vi "Main.vi"() -> ()   [LabVIEW 2017]
doc: "The myRIO Project template acquires acceleration data from the onboard accelerometer and displays the changes of acceleration values in a waveform chart."
uses:
  <vilib>/myRIO/Instrument Drivers/Onboard IO/AI/typedefs/AI Reference.ctl
  <vilib>/myRIO/Common/Instrument Driver Framework/Utilities/typedefs/myRIO Generic Hardware Reference.ctl
  <vilib>/myRIO/Common/Instrument Driver Framework/Utilities/typedefs/Hardware Version Enum.ctl
  <vilib>/myRIO/Common/Instrument Driver Framework/Utilities/typedefs/myRIO v1.0 Reference.ctl
  <vilib>/myRIO/Common/Instrument Driver Framework/Utilities/typedefs/Generic FPGA Reference.ctl
  <vilib>/myRIO/Common/Instrument Driver Framework/myRIO v1.0/AI/typedefs/AI Channels List.ctl
  <vilib>/myRIO/Common/Instrument Driver Framework/myRIO v1.0/AI/typedefs/AI Channels Enum.ctl
  <vilib>/myRIO/Common/Instrument Driver Framework/Utilities/typedefs/Analog Scaling Constants List.ctl
  <vilib>/myRIO/Common/Instrument Driver Framework/Utilities/typedefs/Analog Scaling Constants.ctl
  <vilib>/userdefined/High Color/nirio_resource_hc.ctl
  <vilib>/myRIO/Instrument Drivers/Onboard IO/DIO/typedefs/DIO Reference.ctl
  <vilib>/myRIO/Common/Instrument Driver Framework/myRIO v1.0/DIO/typedefs/DIO Channels List.ctl
  <vilib>/myRIO/Common/Instrument Driver Framework/myRIO v1.0/DIO/typedefs/DIO Channels Enum.ctl
  <vilib>/myRIO/Common/Instrument Driver Framework/Utilities/vis/Is FPGA Ref Available.vi
  <vilib>/myRIO/Common/Instrument Driver Framework/myRIO v1.0/DIO/vis/myRIO v1.1 Open DIO.vi
  <vilib>/myRIO/Instrument Drivers/Onboard IO/DIO/vis/Write.vi
  <vilib>/myRIO/Common/Instrument Driver Framework/myRIO v1.0/AI/vis/myRIO v1.1 Open AI.vi
  <vilib>/myRIO/Instrument Drivers/Onboard IO/AI/vis/Read.vi
  <vilib>/myRIO/Common/Instrument Driver Framework/Utilities/vis/Validate Channels.vi
  <vilib>/myRIO/Common/Instrument Driver Framework/myRIO v1.0/DIO/vis/myRIO v1.0 Reserve DIO.vi
  <vilib>/myRIO/Common/Instrument Driver Framework/myRIO v1.0/AI/vis/myRIO v1.0 Reserve AI.vi
  <vilib>/myRIO/Common/Instrument Driver Framework/myRIO v1.0/Resource Manager/vis/myRIO v1.0 Reserve Channel List.vi
  <vilib>/myRIO/Common/Instrument Driver Framework/myRIO v1.0/DIO/vis/myRIO v1.0 Build MUX Configuration DIO.vi
  <vilib>/myRIO/Common/Instrument Driver Framework/myRIO v1.0/AI/vis/myRIO v1.0 Build MUX Configuration AI.vi
  <vilib>/myRIO/Common/Instrument Driver Framework/myRIO v1.0/Resource Manager/vis/myRIO v1.0 Reserve Channel.vi
  <vilib>/myRIO/Common/Instrument Driver Framework/myRIO v1.0/Resource Manager/vis/myRIO v1.0 Unreserve Channel.vi
  <vilib>/myRIO/Common/Instrument Driver Framework/myRIO v1.0/Resource Manager/vis/myRIO v1.0 Create Configuration List.vi
  <vilib>/myRIO/Common/Instrument Driver Framework/myRIO v1.0/Resource Manager/vis/myRIO v1.0 Build Mutex Name.vi
  GlobalVar.vi
  <vilib>/Utility/VariantDataType/GetNumericInfo.vi
  <vilib>/Utility/error.llb/Error Cluster From Error Code.vi
  <vilib>/myRIO/Common/Instrument Driver Framework/myRIO v1.0/myRIO v1.1 Open.vi
  <vilib>/myRIO/Common/Instrument Driver Framework/myRIO v1.0/AI/vis/myRIO v1.0 Get Scaling Constants AI.vi
  <vilib>/myRIO/Common/Instrument Driver Framework/Utilities/vis/IO Manager.vi
  <vilib>/myRIO/Common/Instrument Driver Framework/Utilities/vis/Configuration Manager.vi
  <vilib>/myRIO/Common/Instrument Driver Framework/myRIO v1.0/myRIO v1.0 Close.vi
  <vilib>/myRIO/Common/Instrument Driver Framework/myRIO v1.0/AI/vis/myRIO v1.0 Read AI.vi
  <vilib>/myRIO/Common/Instrument Driver Framework/myRIO v1.0/Resource Manager/vis/myRIO v1.0 Configure IO.vi
  <vilib>/myRIO/Common/Instrument Driver Framework/myRIO v1.0/DIO/vis/myRIO v1.0 Write DIO.vi
  <vilib>/myRIO/Express VI/Onboard IO/AI/AI Express VI.xnode
  <vilib>/myRIO/Instrument Drivers/Onboard IO/AI/vis/myRIO AI Open.xnode
  <vilib>/myRIO/Express VI/Onboard Devices/LED/LED Express VI.xnode
  <vilib>/myRIO/Instrument Drivers/Onboard IO/DIO/vis/myRIO DIO Open.xnode
  <vilib>/myRIO/Instrument Drivers/Onboard IO/AI/AI.lvlib
  <vilib>/myRIO/Instrument Drivers/Onboard IO/DIO/DIO.lvlib
  <vilib>/myRIO/Express VI/Onboard Devices/Button/Button Express VI.xnode
  <vilib>/myRIO/Instrument Drivers/Onboard IO/DIO/vis/Read.vi
panel:
  in  "x":dbl
  in  "Stop Button 2":bool
  in  "Stop (F)":bool
  out "Image Out":T1(plugin-control)
  in  "Carzeta":dbl
  in  "Stop Button":bool
  out "lb (B/AI3 (Pin 9))":dbl
  out "lf (B/AI2 (Pin 7))":dbl
  out "r (B/AI1 (Pin 5))":dbl
  out "l (B/AI0 (Pin 3))":dbl
  out "L_MOTOR_POS":i32
  out "R_MOTOR_POS":i32
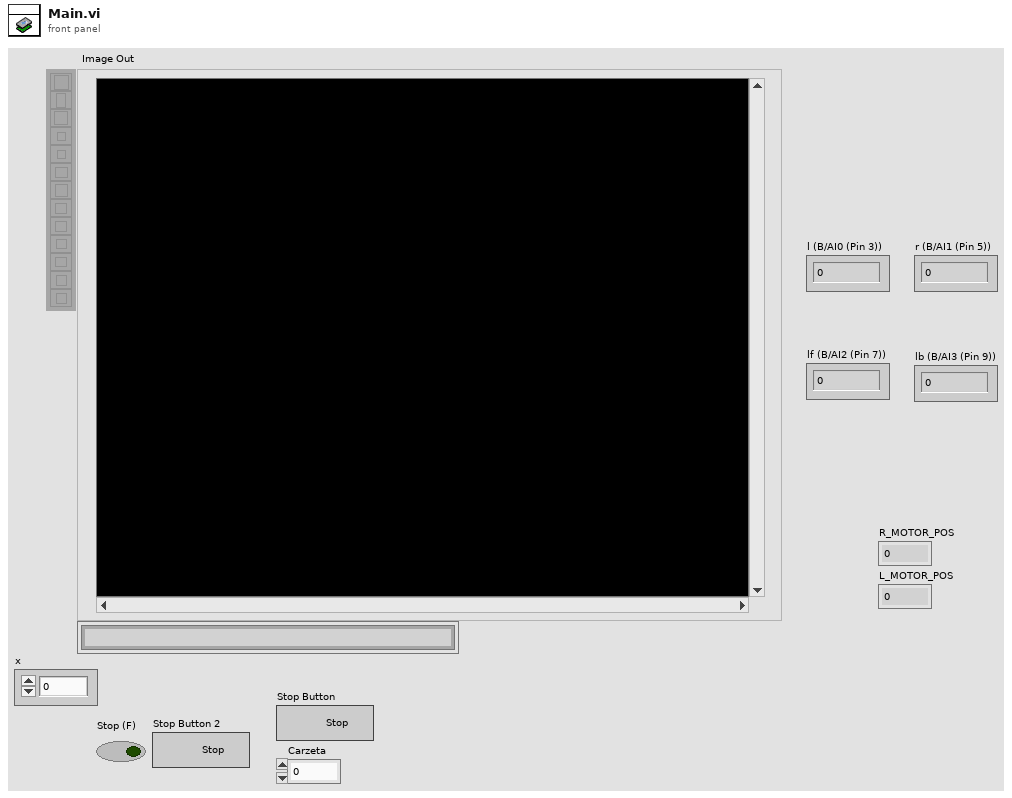
[diagram p1: front panel]
types:
  T1 = typedef "IMAQ Image.ctl" = refnum<image>
  T2 = typedef "AI.lvlib/AI Reference.ctl" = cluster{"myRIO Reference":T3, "AI Channels List":T7, "AI Scaling Constants List":T9}
  T3 = typedef "myRIO Generic Hardware Reference.ctl" = cluster{"myRIO Model":T4, "myRIO Hardware Reference":T5}
  T4 = typedef "Hardware Version Enum.ctl" = enum16{"Unknown", "myRIO-1900", "myRIO-1950", "roboRIO", "NI ELVIS RIO CM"}
  T5 = typedef "myRIO v1.0 Reference.ctl" = cluster{"Generic FPGA Reference":T6, "Allow multiple opens":bool}
  T6 = typedef "Generic FPGA Reference.ctl" = refnum<k20>
  T7 = typedef "AI Channels List.ctl" = T8[]
  T8 = typedef "AI Channels Enum.ctl" = enum16{"Not Connected", "AudioIn/Left", "AudioIn/Right", "C/AI0", "C/AI1", "A/AI0", "A/AI1", "A/AI2", "A/AI3", "B/AI0", "B/AI1", "B/AI2", "B/AI3", "AI/AI0", "AI/AI1", "AI/AI2", "AI/AI3"}
  T9 = typedef "Analog Scaling Constants List.ctl" = T10[]
  T10 = typedef "Analog Scaling Constants.ctl" = cluster{"LSB Weight (Volts)":dbl, "Offset (Volts)":dbl, "Signed?":bool}
  T11 = typedef "nirio_resource_hc.ctl" = tag
  T12 = typedef "DIO.lvlib/DIO Reference.ctl" = cluster{"myRIO Reference":T3, "DIO Channels List":T13}
  T13 = typedef "DIO Channels List.ctl" = T14[]
  T14 = typedef "DIO Channels Enum.ctl" = enum16{"Not Connected", "C/DIO0", "C/DIO1", "C/DIO2", "C/DIO3", "C/DIO4", "C/DIO5", "C/DIO6", "C/DIO7", "A/DIO0", "A/DIO1", "A/DIO2", "A/DIO3", "A/DIO4", "A/DIO5", "A/DIO6", "A/DIO7", "A/DIO8", "A/DIO9", "A/DIO10", "A/DIO11", "A/DIO12", "A/DIO13", "A/DIO14", "A/DIO15", "B/DIO0", "B/DIO1", "B/DIO2", "B/DIO3", "B/DIO4", "B/DIO5", "B/DIO6", "B/DIO7", "B/DIO8", "B/DIO9", "B/DIO10", "B/DIO11", "B/DIO12", "B/DIO13", "B/DIO14", "B/DIO15", "LED0", "LED1", "LED2", "LED3", "Button0", "DIO/DIO0", "DIO/DIO1", "DIO/DIO2", "DIO/DIO3", "DIO/DIO4", "DIO/DIO5", "DIO/DIO6", "DIO/DIO7", "DIO/DIO8", "DIO/DIO9", "SPI/CS0", "SPI/CS1", "SPI/CS2", "SPI/CS3", "LED RADIO (Green)", "LED RADIO (Red)", "LED COMM (Green)", "LED COMM (Red)", "LED MODE (Green)", "LED MODE (Red)"}
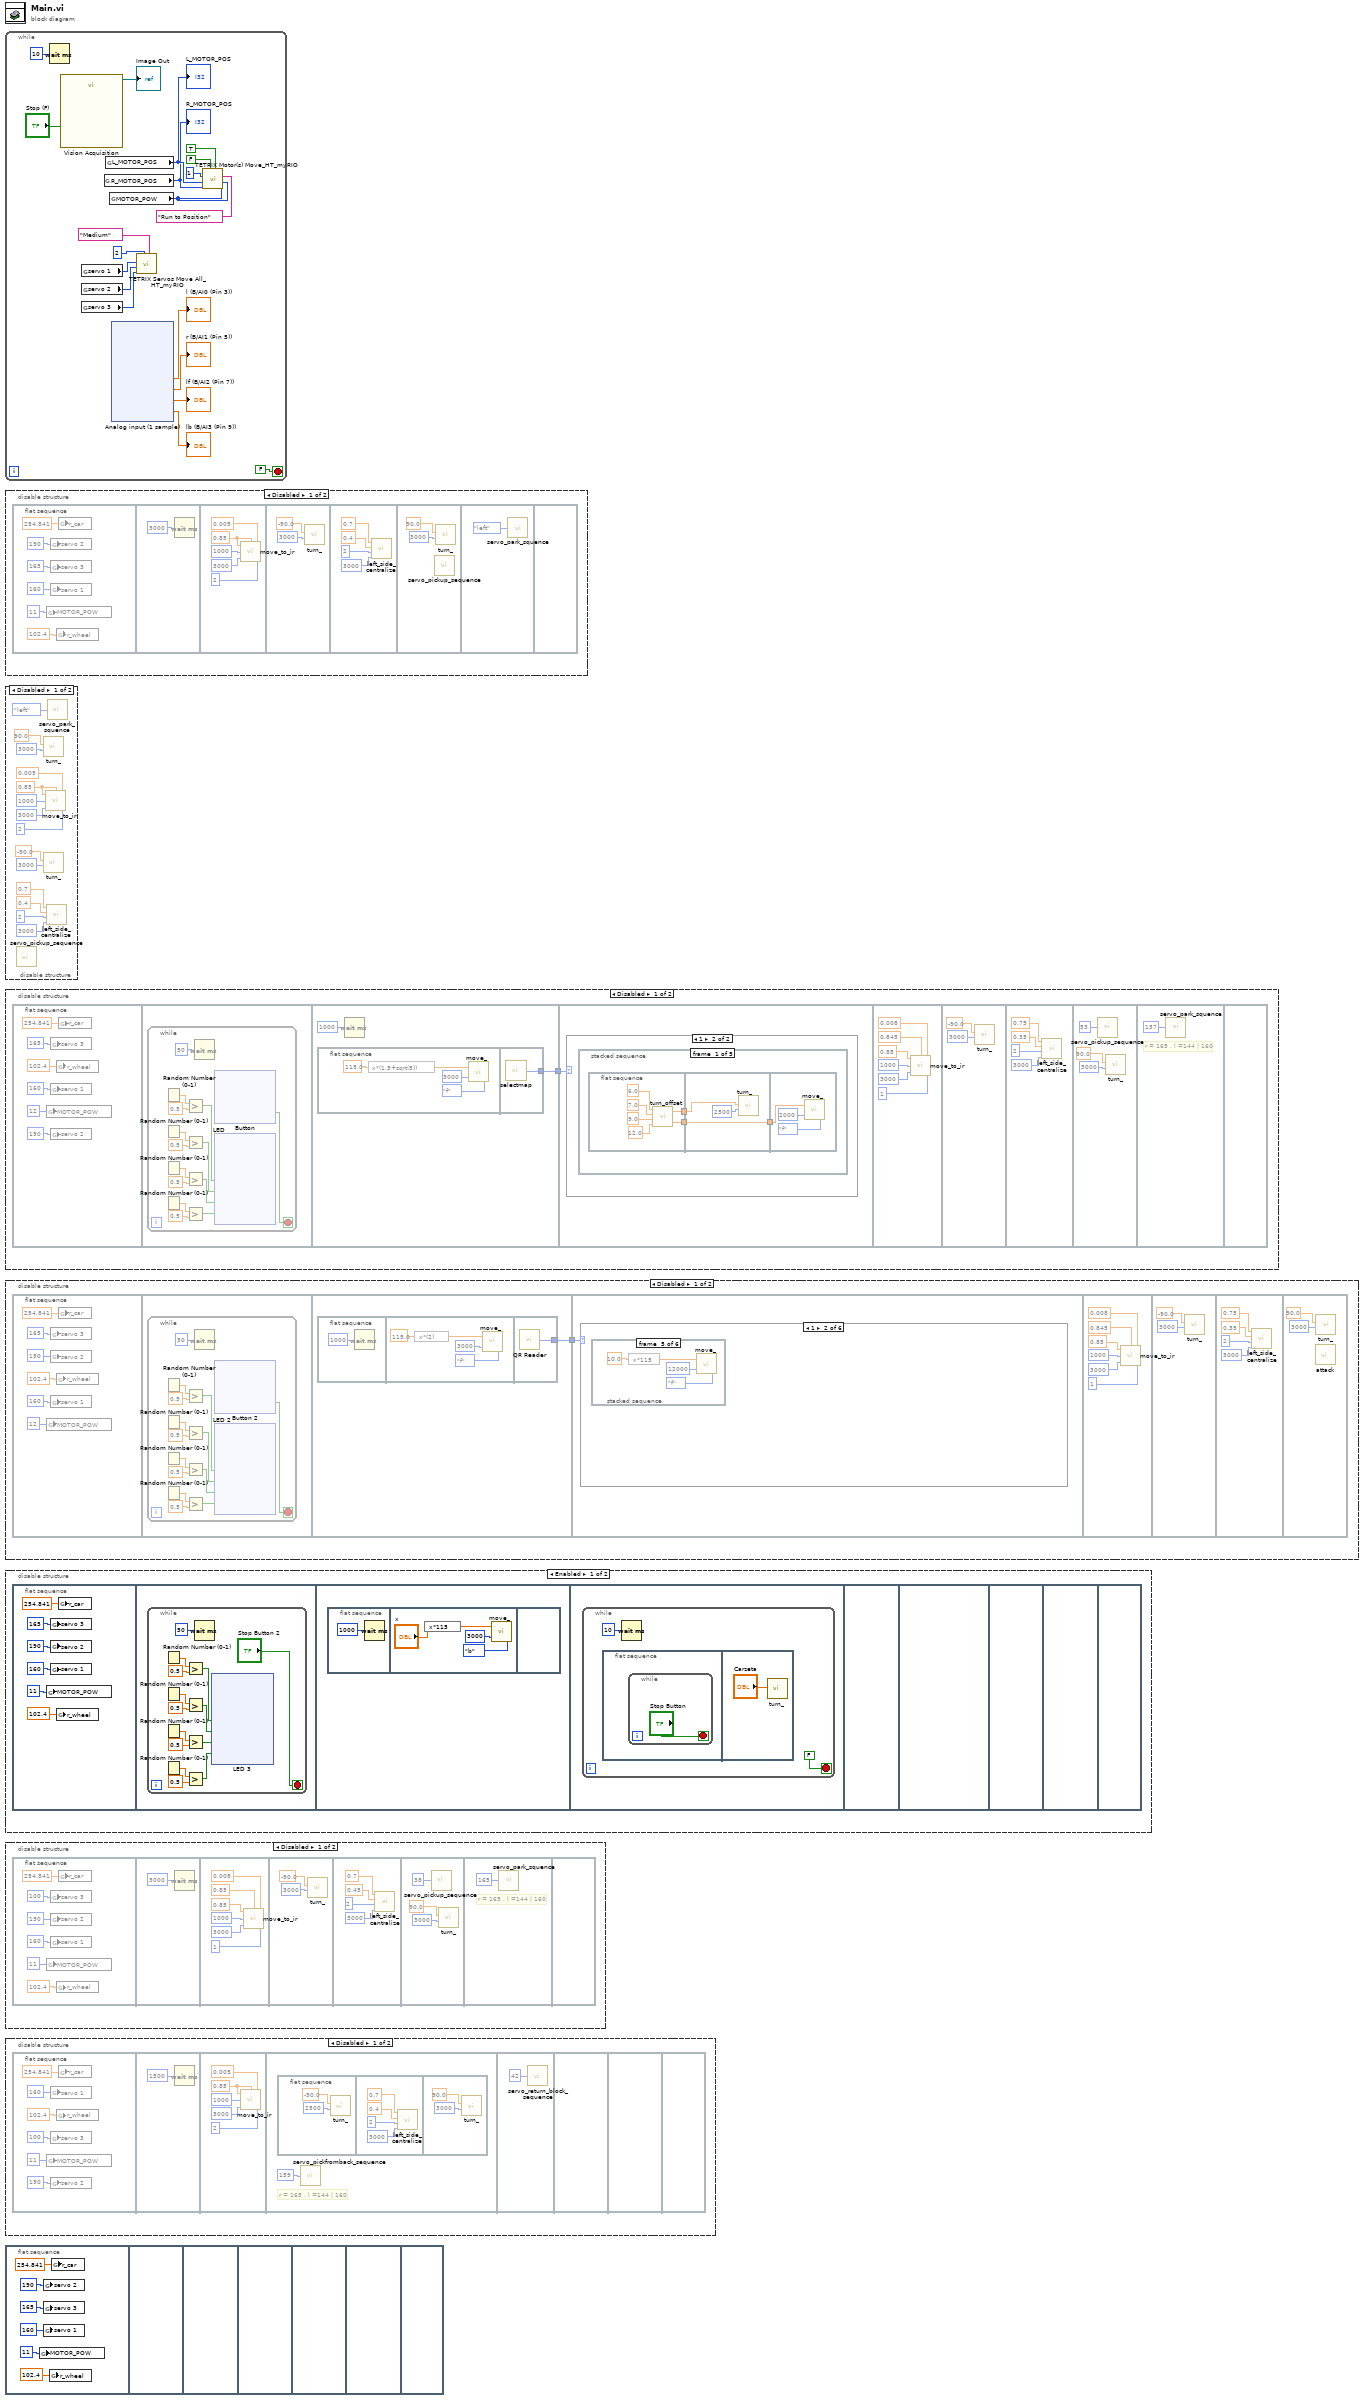
[diagram p0: block diagram]
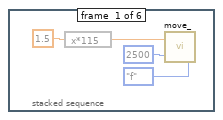
[diagram p3: hidden frame]
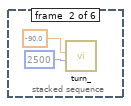
[diagram p4: hidden frame]
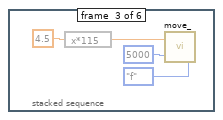
[diagram p5: hidden frame]
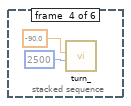
[diagram p6: hidden frame]
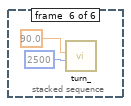
[diagram p7: hidden frame]
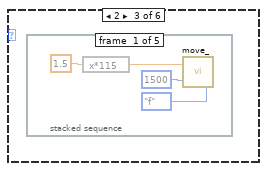
[diagram p8: hidden frame]
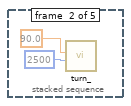
[diagram p9: hidden frame]
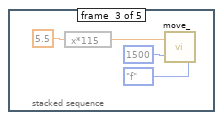
[diagram p10: hidden frame]
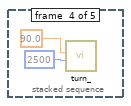
[diagram p11: hidden frame]
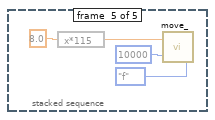
[diagram p12: hidden frame]
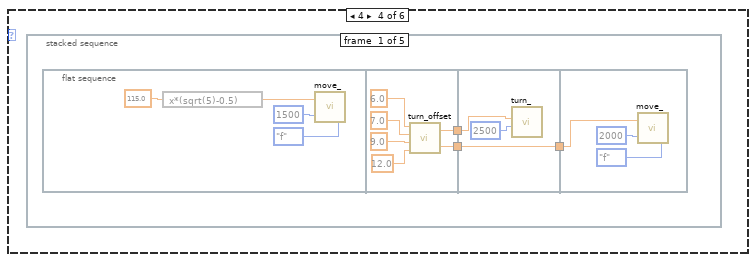
[diagram p13: hidden frame]
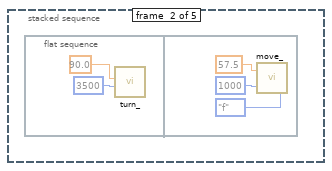
[diagram p14: hidden frame]
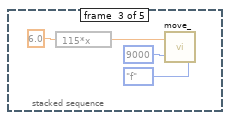
[diagram p15: hidden frame]
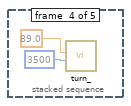
[diagram p16: hidden frame]
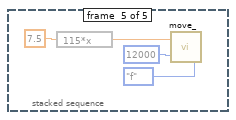
[diagram p17: hidden frame]
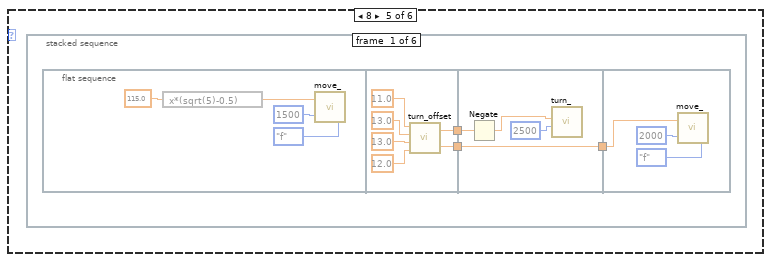
[diagram p18: hidden frame]
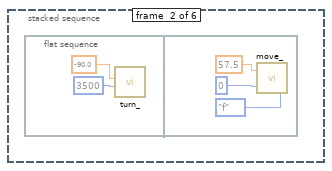
[diagram p19: hidden frame]
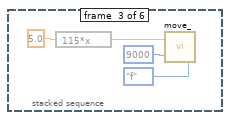
[diagram p20: hidden frame]
diagram:
  n1 = while {
    stop <- FALSE stop-if-true
    n2 = Wait (ms)(milliseconds to wait=u32 10) -> ()  [unwired: 1 out]
    n3 = call "Vision Acquisition"("Stop (F)"="Stop (F)") -> ("Image Out"=→"Image Out":T1)  [unwired: 24 in, 2 out]
    n4 = global read "GlobalVar.vi" "servo 1"() -> (w5:u8)
    n5 = global read "GlobalVar.vi" "servo 2"() -> (w4:u8)
    n6 = global read "GlobalVar.vi" "servo 3"() -> (w3:u8)
    n7 = global read "GlobalVar.vi" "R_MOTOR_POS"() -> (w13:i32)
    "R_MOTOR_POS" <- w13
    n8 = global read "GlobalVar.vi" "L_MOTOR_POS"() -> (w14:i32)
    "L_MOTOR_POS" <- w14
    n9 = global read "GlobalVar.vi" "MOTOR_POW"() -> (w15:i8)
    n10 = xnode "Analog input (1 sample)"() -> ("l (B/AI0 (Pin 3))"=→"l (B/AI0 (Pin 3))":dbl, "r (B/AI1 (Pin 5))"=→"r (B/AI1 (Pin 5))":dbl, "lf (B/AI2 (Pin 7))"=→"lf (B/AI2 (Pin 7))":dbl, "lb (B/AI3 (Pin 9))"=→"lb (B/AI3 (Pin 9))":dbl)  [unwired: 1 in, 1 out]
    n11 = call <vilib>:"TETRIX Servos Move All_HT_myRIO.vi"("Enable Sync: Fast | Medium | Slow | None"="Medium", "Controller Daisy Chain Position (1 - 4)"=u8 2, "Servo 3 (0 - 255)"=w3, "Servo 2 (0 - 255)"=w4, "Servo 1 (0 - 255)"=w5) -> ()  [unwired: 4 in, 1 out]
    n12 = call <vilib>:"TETRIX Motor(s) Move_HT_myRIO.vi"("Motor 2 Power (-100 to 100)\n0 = Stop/Brake\n-128 = Stop/Coast"=w15, "Motor 1 Power (-100 to 100)\n0 = Stop/Brake\n-128 = Stop/Coast"=w15, "Control Mode"="Run to Position", "Motor 2 Reverse? : T or F"=TRUE, "Motor 1 Reverse? : T or F"=FALSE, "Encoder 2 Target: 360 = 1 motor shaft revolution"=w13, "Encoder 1 Target: 360 = 1 motor shaft revolution"=w14, "Controller Daisy Chain Position: 1 - 4"=u8 1) -> ()  [unwired: 1 in, 1 out]
  }
  n13 = disable-structure shown="Disabled" {
    frame Disabled {
      n14 = flat-sequence {
        frame #0 {
          n15 = global write "GlobalVar.vi" "MOTOR_POW"(i8 11 ("MOTOR_POW")) -> ()
          n16 = global write "GlobalVar.vi" "servo 2"(u8 190 ("servo 2")) -> ()
          n17 = global write "GlobalVar.vi" "servo 3"(u8 165 ("servo 3")) -> ()
          n18 = global write "GlobalVar.vi" "servo 1"(u8 160 ("servo 1")) -> ()
          n19 = global write "GlobalVar.vi" "r_wheel"(102.4 ("r_wheel")) -> ()
          n20 = global write "GlobalVar.vi" "r_car"(254.841 ("r_car")) -> ()
        }
        frame #1 {
          n21 = Wait (ms)(milliseconds to wait=u32 3000) -> ()  [unwired: 1 out]
        }
        frame #2 {
          w72 = 0.85 ("target_ir_r")
          n22 = call "move_to_ir.vi"("step"=2, "precision"=0.005, "target_ir_r"=w72, "samples"=3000, "delay_after"=u32 1000, "target_ir_l"=w72) -> ()
        }
        frame #3 {
          n23 = call "turn_.vi"("delay"=u32 3000, "Carzeta"=-90.0) -> ()  [unwired: 10 in]
        }
        frame #4 {
          n24 = call "left_side_centralize.vi"("samples"=3000, "step(mm)"=2, "inner_b_ir"=0.4, "inner_f_ir"=0.7) -> ()
        }
        frame #5 {
          n25 = call "servo_pickup_sequence.vi"() -> ()  [unwired: 12 in]
          n26 = call "turn_.vi"("delay"=u32 3000, "Carzeta"=90.0) -> ()  [unwired: 10 in]
        }
        frame #6 {
          n27 = call "servo_park_squence.vi"("servo 3"=enum16{"left", "right"}."left" ("pos")) -> ()
        }
        frame #7 {
        }
      }
    }
    frame Enabled {
    }
  }
  n28 = disable-structure shown="Disabled" {
    frame Disabled {
      w82 = 0.85 ("target_ir_r")
      n29 = call "servo_pickup_sequence.vi"() -> ()  [unwired: 1 in]
      n30 = call "turn_.vi"("delay"=u32 3000, "Carzeta"=90.0) -> ()  [unwired: 10 in]
      n31 = call "turn_.vi"("delay"=u32 3000, "Carzeta"=-90.0) -> ()  [unwired: 10 in]
      n32 = call "move_to_ir.vi"("step"=2, "precision"=0.005, "target_ir_r"=w82, "samples"=3000, "delay_after"=u32 1000, "target_ir_l"=w82) -> ()
      n33 = call "left_side_centralize.vi"("samples"=3000, "step(mm)"=2, "inner_b_ir"=0.4, "inner_f_ir"=0.7) -> ()
      n34 = call "servo_park_squence.vi"("servo 3"=enum16{"left", "right"}."left" ("pos")) -> ()
    }
    frame Enabled {
    }
  }
  n35 = disable-structure shown="Disabled" {
    frame Disabled {
      n36 = flat-sequence {
        tunnel: [w190] -> w96
        tunnel: w96 -> [w197]
        frame #0 {
          n37 = global write "GlobalVar.vi" "MOTOR_POW"(i8 12 ("MOTOR_POW")) -> ()
          n38 = global write "GlobalVar.vi" "servo 3"(u8 165 ("servo 3")) -> ()
          n39 = global write "GlobalVar.vi" "servo 1"(u8 160 ("servo 1")) -> ()
          n40 = global write "GlobalVar.vi" "servo 2"(u8 190 ("servo 2")) -> ()
          n41 = global write "GlobalVar.vi" "r_wheel"(102.4 ("r_wheel")) -> ()
          n42 = global write "GlobalVar.vi" "r_car"(254.841 ("r_car")) -> ()
        }
        frame #1 {
          n43 = while {
            stop <- w103 stop-if-true
            n44 = Random Number (0-1)() -> (number: 0 to 1=w108:dbl)
            n45 = Random Number (0-1)() -> (number: 0 to 1=w115:dbl)
            n46 = Random Number (0-1)() -> (number: 0 to 1=w112:dbl)
            n47 = Random Number (0-1)() -> (number: 0 to 1=w111:dbl)
            n48 = Greater?(x=w108, y=0.5) -> (0:w107:bool)
            n49 = Greater?(x=w115, y=0.5) -> (0:w106:bool)
            n50 = Greater?(x=w112, y=0.5) -> (0:w105:bool)
            n51 = Greater?(x=w111, y=0.5) -> (0:w104:bool)
            n52 = Wait (ms)(milliseconds to wait=u32 50) -> ()  [unwired: 1 out]
            n53 = xnode "Button"() -> ("Value"=w103:bool)  [unwired: 1 in, 1 out]
            n54 = xnode "LED"("LED0"=w107, "LED1"=w106, "LED2"=w105, "LED3"=w104) -> ()  [unwired: 1 in, 1 out]
          }
        }
        frame #2 {
          n55 = flat-sequence {
            tunnel: [w196] -> w190
            frame #0 {
              n56 = expression code="x*(1.5+sqrt(5))"(115.0 ("x")) -> (w195:dbl)
              n57 = call "move_.vi"("Enum"=enum16{"hold", "f", "b"}."f", "delay"=u32 3000, "D"=w195) -> ()  [unwired: 1 in]
            }
            frame #1 {
              n58 = call "selectmap.vi"() -> ("binary"=w196:u32)
            }
          }
          n59 = Wait (ms)(milliseconds to wait=u32 1000) -> ()  [unwired: 1 out]
        }
        frame #3 {
          n60 = case shown="1" w197 {
            frame 0, Default {
            }
            frame 1 {
              n61 = stacked-sequence {
                frame #0 {
                  n62 = flat-sequence {
                    tunnel: [w202] -> w200
                    tunnel: [w201] -> w198
                    tunnel: w200 -> [w208]
                    tunnel: [w207] -> w199
                    tunnel: w198 -> [w207]
                    tunnel: w199 -> [w210]
                    frame #0 {
                      n63 = call "turn_offset.vi"("x2"=12.0, "x1"=9.0, "y2"=7.0, "y1"=6.0) -> ("dis_"=w201:dbl, "zeta"=w202:dbl)
                    }
                    frame #1 {
                      n64 = call "turn_.vi"("delay"=u32 2500, "Carzeta"=w208) -> ()  [unwired: 10 in]
                    }
                    frame #2 {
                      n65 = call "move_.vi"("Enum"=enum16{"hold", "f", "b"}."f", "delay"=u32 2000, "D"=w210) -> ()  [unwired: 1 in]
                    }
                  }
                }
                frame #1 {
                  n66 = flat-sequence {
                    frame #0 {
                      n67 = call "turn_.vi"("delay"=u32 3500, "Carzeta"=90.0) -> ()  [unwired: 10 in]
                    }
                    frame #1 {
                      n68 = call "move_.vi"("Enum"=enum16{"hold", "f", "b"}."f", "delay"=u32 1000, "D"=57.5) -> ()  [unwired: 1 in]
                    }
                  }
                }
                frame #2 {
                  n69 = expression code="115*x"(6.0) -> (w221:dbl)
                  n70 = call "move_.vi"("Enum"=enum16{"hold", "f", "b"}."f", "delay"=u32 9000, "D"=w221) -> ()  [unwired: 1 in]
                }
                frame #3 {
                  n71 = call "turn_.vi"("delay"=u32 3500, "Carzeta"=89.0) -> ()  [unwired: 10 in]
                }
                frame #4 {
                  n72 = expression code="115*x"(7.5) -> (w227:dbl)
                  n73 = call "move_.vi"("Enum"=enum16{"hold", "f", "b"}."f", "delay"=u32 12000, "D"=w227) -> ()  [unwired: 1 in]
                }
              }
            }
          }
        }
        frame #4 {
          n74 = call "move_to_ir.vi"("step"=1, "precision"=0.008, "target_ir_r"=0.845, "samples"=3000, "delay_after"=u32 1000, "target_ir_l"=0.85 ("target_ir_r")) -> ()
        }
        frame #5 {
          n75 = call "turn_.vi"("delay"=u32 3000, "Carzeta"=-90.0) -> ()  [unwired: 10 in]
        }
        frame #6 {
          n76 = call "left_side_centralize.vi"("samples"=3000, "step(mm)"=2, "inner_b_ir"=0.35, "inner_f_ir"=0.75) -> ()
        }
        frame #7 {
          n77 = call "servo_pickup_sequence.vi"("servo 3"=u8 53) -> ()
          n78 = call "turn_.vi"("delay"=u32 3000, "Carzeta"=90.0) -> ()  [unwired: 10 in]
        }
        frame #8 {
          # "r = 165 , l =144 | 160"
          n79 = call "servo_park_squence.vi"("servo 3"=u8 157) -> ()
        }
        frame #9 {
        }
      }
    }
    frame Enabled {
    }
  }
  n80 = disable-structure shown="Disabled" {
    frame Disabled {
      n81 = flat-sequence {
        tunnel: [w338] -> w244
        tunnel: w244 -> [w345]
        frame #0 {
          n82 = global write "GlobalVar.vi" "MOTOR_POW"(i8 12 ("MOTOR_POW")) -> ()
          n83 = global write "GlobalVar.vi" "servo 3"(u8 165 ("servo 3")) -> ()
          n84 = global write "GlobalVar.vi" "servo 2"(u8 190 ("servo 2")) -> ()
          n85 = global write "GlobalVar.vi" "servo 1"(u8 160 ("servo 1")) -> ()
          n86 = global write "GlobalVar.vi" "r_wheel"(102.4 ("r_wheel")) -> ()
          n87 = global write "GlobalVar.vi" "r_car"(254.841 ("r_car")) -> ()
        }
        frame #1 {
          n88 = while {
            stop <- w251 stop-if-true
            n89 = Random Number (0-1)() -> (number: 0 to 1=w256:dbl)
            n90 = Random Number (0-1)() -> (number: 0 to 1=w263:dbl)
            n91 = Random Number (0-1)() -> (number: 0 to 1=w260:dbl)
            n92 = Random Number (0-1)() -> (number: 0 to 1=w259:dbl)
            n93 = Greater?(x=w256, y=0.5) -> (0:w255:bool)
            n94 = Greater?(x=w263, y=0.5) -> (0:w254:bool)
            n95 = Greater?(x=w260, y=0.5) -> (0:w253:bool)
            n96 = Greater?(x=w259, y=0.5) -> (0:w252:bool)
            n97 = Wait (ms)(milliseconds to wait=u32 50) -> ()  [unwired: 1 out]
            n98 = xnode "Button 2"() -> ("Value"=w251:bool)  [unwired: 1 in, 1 out]
            n99 = xnode "LED 2"("LED0"=w255, "LED1"=w254, "LED2"=w253, "LED3"=w252) -> ()  [unwired: 1 in, 1 out]
          }
        }
        frame #2 {
          n100 = flat-sequence {
            tunnel: [w344] -> w338
            frame #0 {
              n101 = Wait (ms)(milliseconds to wait=u32 1000) -> ()  [unwired: 1 out]
            }
            frame #1 {
              n102 = expression code="x*(2)"(115.0 ("x")) -> (w343:dbl)
              n103 = call "move_.vi"("Enum"=enum16{"hold", "f", "b"}."f", "delay"=u32 3000, "D"=w343) -> ()  [unwired: 1 in]
            }
            frame #2 {
              n104 = call "QR Reader.vi"() -> ("eiei"=w344:u32)
            }
          }
        }
        frame #3 {
          n105 = case shown="1" w345 {
            frame 0, Default {
            }
            frame 1 {
              n106 = stacked-sequence {
                frame #0 {
                  n107 = expression code="x*115"(1.5 ("x")) -> (w346:dbl)
                  n108 = call "move_.vi"("Enum"=enum16{"hold", "f", "b"}."f", "delay"=u32 2500, "D"=w346) -> ()  [unwired: 1 in]
                }
                frame #1 {
                  n109 = call "turn_.vi"("delay"=u32 2500, "Carzeta"=-90.0) -> ()  [unwired: 10 in]
                }
                frame #2 {
                  n110 = expression code="x*115"(4.5 ("x")) -> (w352:dbl)
                  n111 = call "move_.vi"("Enum"=enum16{"hold", "f", "b"}."f", "delay"=u32 5000, "D"=w352) -> ()  [unwired: 1 in]
                }
                frame #3 {
                  n112 = call "turn_.vi"("delay"=u32 2500, "Carzeta"=-90.0) -> ()  [unwired: 10 in]
                }
                frame #4 {
                  n113 = expression code="x*115"(10.0 ("x")) -> (w358:dbl)
                  n114 = call "move_.vi"("Enum"=enum16{"hold", "f", "b"}."f", "delay"=u32 12000, "D"=w358) -> ()  [unwired: 1 in]
                }
                frame #5 {
                  n115 = call "turn_.vi"("delay"=u32 2500, "Carzeta"=90.0) -> ()  [unwired: 10 in]
                }
              }
            }
            frame 2 {
              n116 = stacked-sequence {
                frame #0 {
                  n117 = expression code="x*115"(1.5 ("x")) -> (w364:dbl)
                  n118 = call "move_.vi"("Enum"=enum16{"hold", "f", "b"}."f", "delay"=u32 1500, "D"=w364) -> ()  [unwired: 1 in]
                }
                frame #1 {
                  n119 = call "turn_.vi"("delay"=u32 2500, "Carzeta"=90.0) -> ()  [unwired: 10 in]
                }
                frame #2 {
                  n120 = expression code="x*115"(5.5 ("x")) -> (w370:dbl)
                  n121 = call "move_.vi"("Enum"=enum16{"hold", "f", "b"}."f", "delay"=u32 1500, "D"=w370) -> ()  [unwired: 1 in]
                }
                frame #3 {
                  n122 = call "turn_.vi"("delay"=u32 2500, "Carzeta"=90.0) -> ()  [unwired: 10 in]
                }
                frame #4 {
                  n123 = expression code="x*115"(8.0 ("x")) -> (w376:dbl)
                  n124 = call "move_.vi"("Enum"=enum16{"hold", "f", "b"}."f", "delay"=u32 10000, "D"=w376) -> ()  [unwired: 1 in]
                }
              }
            }
            frame 4 {
              n125 = stacked-sequence {
                frame #0 {
                  n126 = flat-sequence {
                    tunnel: [w388] -> w382
                    tunnel: [w387] -> w380
                    tunnel: w382 -> [w394]
                    tunnel: [w393] -> w381
                    tunnel: w380 -> [w393]
                    tunnel: w381 -> [w396]
                    frame #0 {
                      n127 = expression code="x*(sqrt(5)-0.5)"(115.0 ("x")) -> (w385:dbl)
                      n128 = call "move_.vi"("Enum"=enum16{"hold", "f", "b"}."f", "delay"=u32 1500, "D"=w385) -> ()  [unwired: 1 in]
                    }
                    frame #1 {
                      n129 = call "turn_offset.vi"("x2"=12.0, "x1"=9.0, "y2"=7.0, "y1"=6.0) -> ("dis_"=w387:dbl, "zeta"=w388:dbl)
                    }
                    frame #2 {
                      n130 = call "turn_.vi"("delay"=u32 2500, "Carzeta"=w394) -> ()  [unwired: 10 in]
                    }
                    frame #3 {
                      n131 = call "move_.vi"("Enum"=enum16{"hold", "f", "b"}."f", "delay"=u32 2000, "D"=w396) -> ()  [unwired: 1 in]
                    }
                  }
                }
                frame #1 {
                  n132 = flat-sequence {
                    frame #0 {
                      n133 = call "turn_.vi"("delay"=u32 3500, "Carzeta"=90.0) -> ()  [unwired: 10 in]
                    }
                    frame #1 {
                      n134 = call "move_.vi"("Enum"=enum16{"hold", "f", "b"}."f", "delay"=u32 1000, "D"=57.5) -> ()  [unwired: 1 in]
                    }
                  }
                }
                frame #2 {
                  n135 = expression code="115*x"(6.0) -> (w407:dbl)
                  n136 = call "move_.vi"("Enum"=enum16{"hold", "f", "b"}."f", "delay"=u32 9000, "D"=w407) -> ()  [unwired: 1 in]
                }
                frame #3 {
                  n137 = call "turn_.vi"("delay"=u32 3500, "Carzeta"=89.0) -> ()  [unwired: 10 in]
                }
                frame #4 {
                  n138 = expression code="115*x"(7.5) -> (w413:dbl)
                  n139 = call "move_.vi"("Enum"=enum16{"hold", "f", "b"}."f", "delay"=u32 12000, "D"=w413) -> ()  [unwired: 1 in]
                }
              }
            }
            frame 8 {
              n140 = stacked-sequence {
                frame #0 {
                  n141 = flat-sequence {
                    tunnel: [w422] -> w416
                    tunnel: [w421] -> w414
                    tunnel: w416 -> [w427]
                    tunnel: [w429] -> w415
                    tunnel: w414 -> [w429]
                    tunnel: w415 -> [w431]
                    frame #0 {
                      n142 = expression code="x*(sqrt(5)-0.5)"(115.0 ("x")) -> (w419:dbl)
                      n143 = call "move_.vi"("Enum"=enum16{"hold", "f", "b"}."f", "delay"=u32 1500, "D"=w419) -> ()  [unwired: 1 in]
                    }
                    frame #1 {
                      n144 = call "turn_offset.vi"("x2"=12.0, "x1"=13.0, "y2"=13.0, "y1"=11.0) -> ("dis_"=w421:dbl, "zeta"=w422:dbl)
                    }
                    frame #2 {
                      n145 = Negate(x=w427) -> (-x=w428:dbl)
                      n146 = call "turn_.vi"("delay"=u32 2500, "Carzeta"=w428) -> ()  [unwired: 10 in]
                    }
                    frame #3 {
                      n147 = call "move_.vi"("Enum"=enum16{"hold", "f", "b"}."f", "delay"=u32 2000, "D"=w431) -> ()  [unwired: 1 in]
                    }
                  }
                }
                frame #1 {
                  n148 = flat-sequence {
                    frame #0 {
                      n149 = call "turn_.vi"("delay"=u32 3500, "Carzeta"=-90.0) -> ()  [unwired: 10 in]
                    }
                    frame #1 {
                      n150 = call "move_.vi"("Enum"=enum16{"hold", "f", "b"}."f", "delay"=u32 0, "D"=57.5) -> ()  [unwired: 1 in]
                    }
                  }
                }
                frame #2 {
                  n151 = expression code="115*x"(5.0) -> (w442:dbl)
                  n152 = call "move_.vi"("Enum"=enum16{"hold", "f", "b"}."f", "delay"=u32 9000, "D"=w442) -> ()  [unwired: 1 in]
                }
                frame #3 {
                  n153 = call "turn_.vi"("delay"=u32 3500, "Carzeta"=-90.0) -> ()  [unwired: 10 in]
                }
                frame #4 {
                  n154 = expression code="115*x"(7.5) -> (w448:dbl)
                  n155 = call "move_.vi"("Enum"=enum16{"hold", "f", "b"}."f", "delay"=u32 12000, "D"=w448) -> ()  [unwired: 1 in]
                }
                frame #5 {
                  n156 = flat-sequence {
                    frame #0 {
                      n157 = call "turn_.vi"("delay"=u32 3000, "Carzeta"=90.0) -> ()  [unwired: 10 in]
                    }
                  }
                }
              }
            }
            frame 16 {
              n158 = stacked-sequence {
                frame #0 {
                  n159 = flat-sequence {
                    tunnel: [w459] -> w453
                    tunnel: [w458] -> w451
                    tunnel: w453 -> [w464]
                    tunnel: [w466] -> w452
                    tunnel: w451 -> [w466]
                    tunnel: w452 -> [w468]
                    frame #0 {
                      n160 = expression code="x*(sqrt(5)-0.5)"(115.0 ("x")) -> (w456:dbl)
                      n161 = call "move_.vi"("Enum"=enum16{"hold", "f", "b"}."f", "delay"=u32 1500, "D"=w456) -> ()  [unwired: 1 in]
                    }
                    frame #1 {
                      n162 = call "turn_offset.vi"("x2"=12.0, "x1"=10.0, "y2"=15.0, "y1"=16.0) -> ("dis_"=w458:dbl, "zeta"=w459:dbl)
                    }
                    frame #2 {
                      n163 = Negate(x=w464) -> (-x=w465:dbl)
                      n164 = call "turn_.vi"("delay"=u32 2500, "Carzeta"=w465) -> ()  [unwired: 10 in]
                    }
                    frame #3 {
                      n165 = call "move_.vi"("Enum"=enum16{"hold", "f", "b"}."f", "delay"=u32 2000, "D"=w468) -> ()  [unwired: 1 in]
                    }
                  }
                }
                frame #1 {
                  n166 = flat-sequence {
                    frame #0 {
                      n167 = call "turn_.vi"("delay"=u32 3500, "Carzeta"=-90.0) -> ()  [unwired: 10 in]
                    }
                    frame #1 {
                      n168 = call "move_.vi"("Enum"=enum16{"hold", "f", "b"}."f", "delay"=u32 0, "D"=57.5) -> ()  [unwired: 1 in]
                    }
                  }
                }
                frame #2 {
                  n169 = expression code="115*x"(6.0) -> (w479:dbl)
                  n170 = call "move_.vi"("Enum"=enum16{"hold", "f", "b"}."f", "delay"=u32 9000, "D"=w479) -> ()  [unwired: 1 in]
                }
                frame #3 {
                  n171 = call "turn_.vi"("delay"=u32 3500, "Carzeta"=90.0) -> ()  [unwired: 10 in]
                }
                frame #4 {
                  n172 = expression code="115*x"(1.0) -> (w485:dbl)
                  n173 = call "move_.vi"("Enum"=enum16{"hold", "f", "b"}."f", "delay"=u32 1500, "D"=w485) -> ()  [unwired: 1 in]
                }
                frame #5 {
                  n174 = flat-sequence {
                    frame #0 {
                      n175 = call "turn_.vi"("delay"=u32 3000, "Carzeta"=-90.0) -> ()  [unwired: 10 in]
                    }
                  }
                }
              }
            }
          }
        }
        frame #4 {
          n176 = call "move_to_ir.vi"("step"=1, "precision"=0.008, "target_ir_r"=0.845, "samples"=3000, "delay_after"=u32 1000, "target_ir_l"=0.85 ("target_ir_r")) -> ()
        }
        frame #5 {
          n177 = call "turn_.vi"("delay"=u32 3000, "Carzeta"=-90.0) -> ()  [unwired: 10 in]
        }
        frame #6 {
          n178 = call "left_side_centralize.vi"("samples"=3000, "step(mm)"=2, "inner_b_ir"=0.35, "inner_f_ir"=0.75) -> ()
        }
        frame #7 {
          n179 = call "attack.vi"() -> ()  [unwired: 12 in]
          n180 = call "turn_.vi"("delay"=u32 3000, "Carzeta"=90.0) -> ()  [unwired: 10 in]
        }
      }
    }
    frame Enabled {
    }
  }
  n181 = disable-structure shown="Enabled" {
    frame Enabled {
      n182 = flat-sequence {
        frame #0 {
          n183 = global write "GlobalVar.vi" "MOTOR_POW"(i8 11 ("MOTOR_POW")) -> ()
          n184 = global write "GlobalVar.vi" "servo 3"(u8 165 ("servo 3")) -> ()
          n185 = global write "GlobalVar.vi" "servo 2"(u8 190 ("servo 2")) -> ()
          n186 = global write "GlobalVar.vi" "servo 1"(u8 160 ("servo 1")) -> ()
          n187 = global write "GlobalVar.vi" "r_wheel"(102.4 ("r_wheel")) -> ()
          n188 = global write "GlobalVar.vi" "r_car"(254.841 ("r_car")) -> ()
        }
        frame #1 {
          n189 = while {
            stop <- "Stop Button 2" stop-if-true
            n190 = Random Number (0-1)() -> (number: 0 to 1=w513:dbl)
            n191 = Random Number (0-1)() -> (number: 0 to 1=w520:dbl)
            n192 = Random Number (0-1)() -> (number: 0 to 1=w517:dbl)
            n193 = Random Number (0-1)() -> (number: 0 to 1=w516:dbl)
            n194 = Greater?(x=w513, y=0.5) -> (0:w512:bool)
            n195 = Greater?(x=w520, y=0.5) -> (0:w511:bool)
            n196 = Greater?(x=w517, y=0.5) -> (0:w510:bool)
            n197 = Greater?(x=w516, y=0.5) -> (0:w509:bool)
            n198 = Wait (ms)(milliseconds to wait=u32 50) -> ()  [unwired: 1 out]
            n199 = xnode "LED 3"("LED0"=w512, "LED1"=w511, "LED2"=w510, "LED3"=w509) -> ()  [unwired: 1 in, 1 out]
          }
        }
        frame #2 {
          n200 = flat-sequence {
            frame #0 {
              n201 = Wait (ms)(milliseconds to wait=u32 1000) -> ()  [unwired: 1 out]
            }
            frame #1 {
              n202 = expression code="x*115"("x") -> (w564:dbl)
              n203 = call "move_.vi"("Enum"=enum16{"hold", "f", "b"}."b", "delay"=u32 3000, "D"=w564) -> ()  [unwired: 1 in]
            }
            frame #2 {
            }
          }
        }
        frame #3 {
          n204 = while {
            stop <- FALSE stop-if-true
            n205 = flat-sequence {
              frame #0 {
                n206 = while {
                  stop <- "Stop Button" stop-if-true
                }
              }
              frame #1 {
                n207 = call "turn_.vi"("Carzeta"="Carzeta") -> ()  [unwired: 11 in]
              }
            }
            n208 = Wait (ms)(milliseconds to wait=u32 10) -> ()  [unwired: 1 out]
          }
        }
        frame #4 {
        }
        frame #5 {
        }
        frame #6 {
        }
        frame #7 {
        }
        frame #8 {
        }
      }
    }
    frame Disabled {
    }
  }
  n209 = disable-structure shown="Disabled" {
    frame Disabled {
      n210 = flat-sequence {
        frame #0 {
          n211 = global write "GlobalVar.vi" "MOTOR_POW"(i8 11 ("MOTOR_POW")) -> ()
          n212 = global write "GlobalVar.vi" "servo 3"(u8 100 ("servo 3")) -> ()
          n213 = global write "GlobalVar.vi" "servo 2"(u8 190 ("servo 2")) -> ()
          n214 = global write "GlobalVar.vi" "servo 1"(u8 160 ("servo 1")) -> ()
          n215 = global write "GlobalVar.vi" "r_wheel"(102.4 ("r_wheel")) -> ()
          n216 = global write "GlobalVar.vi" "r_car"(254.841 ("r_car")) -> ()
        }
        frame #1 {
          n217 = Wait (ms)(milliseconds to wait=u32 3000) -> ()  [unwired: 1 out]
        }
        frame #2 {
          n218 = call "move_to_ir.vi"("step"=1, "precision"=0.008, "target_ir_r"=0.85, "samples"=3000, "delay_after"=u32 1000, "target_ir_l"=0.85 ("target_ir_r")) -> ()
        }
        frame #3 {
          n219 = call "turn_.vi"("delay"=u32 3000, "Carzeta"=-90.0) -> ()  [unwired: 10 in]
        }
        frame #4 {
          n220 = call "left_side_centralize.vi"("samples"=3000, "step(mm)"=2, "inner_b_ir"=0.45, "inner_f_ir"=0.7) -> ()
        }
        frame #5 {
          n221 = call "servo_pickup_sequence.vi"("servo 3"=u8 38) -> ()
          n222 = call "turn_.vi"("delay"=u32 3000, "Carzeta"=90.0) -> ()  [unwired: 10 in]
        }
        frame #6 {
          # "r = 165 , l =144 | 160"
          n223 = call "servo_park_squence.vi"("servo 3"=u8 165) -> ()
        }
        frame #7 {
        }
      }
    }
    frame Enabled {
    }
  }
  n224 = disable-structure shown="Disabled" {
    frame Disabled {
      n225 = flat-sequence {
        frame #0 {
          n226 = global write "GlobalVar.vi" "MOTOR_POW"(i8 11 ("MOTOR_POW")) -> ()
          n227 = global write "GlobalVar.vi" "servo 1"(u8 160 ("servo 1")) -> ()
          n228 = global write "GlobalVar.vi" "servo 3"(u8 100 ("servo 3")) -> ()
          n229 = global write "GlobalVar.vi" "servo 2"(u8 190 ("servo 2")) -> ()
          n230 = global write "GlobalVar.vi" "r_wheel"(102.4 ("r_wheel")) -> ()
          n231 = global write "GlobalVar.vi" "r_car"(254.841 ("r_car")) -> ()
        }
        frame #1 {
          n232 = Wait (ms)(milliseconds to wait=u32 1500) -> ()  [unwired: 1 out]
        }
        frame #2 {
          w603 = 0.85 ("target_ir_r")
          n233 = call "move_to_ir.vi"("step"=2, "precision"=0.005, "target_ir_r"=w603, "samples"=3000, "delay_after"=u32 1000, "target_ir_l"=w603) -> ()
        }
        frame #3 {
          # "r = 165 , l =144 | 160"
          n234 = flat-sequence {
            frame #0 {
              n235 = call "turn_.vi"("delay"=u32 2500, "Carzeta"=-90.0) -> ()  [unwired: 10 in]
            }
            frame #1 {
              n236 = call "left_side_centralize.vi"("samples"=3000, "step(mm)"=2, "inner_b_ir"=0.4, "inner_f_ir"=0.7) -> ()
            }
            frame #2 {
              n237 = call "turn_.vi"("delay"=u32 3000, "Carzeta"=90.0) -> ()  [unwired: 10 in]
            }
          }
          n238 = call "servo_pickfromback_sequence.vi"("servo 3"=u8 159) -> ()
        }
        frame #4 {
          n239 = call "servo_return_block_sequence.vi"("servo 3"=u8 42) -> ()
        }
        frame #5 {
        }
        frame #6 {
        }
        frame #7 {
        }
      }
    }
    frame Enabled {
    }
  }
  n240 = flat-sequence {
    frame #0 {
      n241 = global write "GlobalVar.vi" "MOTOR_POW"(i8 11 ("MOTOR_POW")) -> ()
      n242 = global write "GlobalVar.vi" "servo 2"(u8 190 ("servo 2")) -> ()
      n243 = global write "GlobalVar.vi" "servo 3"(u8 165 ("servo 3")) -> ()
      n244 = global write "GlobalVar.vi" "servo 1"(u8 160 ("servo 1")) -> ()
      n245 = global write "GlobalVar.vi" "r_wheel"(102.4 ("r_wheel")) -> ()
      n246 = global write "GlobalVar.vi" "r_car"(254.841 ("r_car")) -> ()
    }
    frame #1 {
    }
    frame #2 {
    }
    frame #3 {
    }
    frame #4 {
    }
    frame #5 {
    }
    frame #6 {
    }
  }
